vi "Get_State.vi"(11 "State Array In":string[](array[string])) -> (3 "State Array Out":string[](array[string]), 5 "Current State":string)   [LabVIEW 2010]
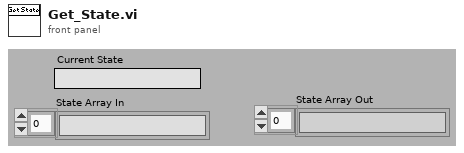
[diagram p1: front panel]
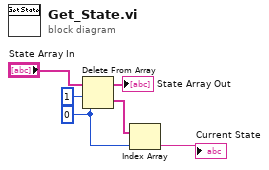
[diagram p0: block diagram]
diagram:
  w5 = 0 ("index")
  n1 = Delete From Array(array="State Array In", length=1, index=w5) -> (deleted portion=w4:string[], array with subset deleted=→"State Array Out":string[])
  n2 = Index Array(array=w4, index=w5) -> (element=→"Current State":string)
